vi "StepUI.vi"() -> ()   [LabVIEW 2015, in "StepNode.lvclass"]
doc: "Copyright 2017 National Instruments Corporation\n\nLicensed under the Apache License, Version 2.0 (the \"License\"); you may not use this file except in compliance with the License. You may obtain a copy of the License at http://www.apache.org/licenses/LICENSE-2.0\nUnless required by applicable law or agreed to in writing, software distributed under the License is distributed on an \"AS IS\" BASIS, WITHOUT WARRANTIES OR CONDITIONS OF ANY KIND, either express or implied. See the License for the specific language governing permissions and limitations under the License."
uses:
  StepNode.lvclass
  <vilib>/NI/Configuration Framework/Node/NodeRef.ctl
  <vilib>/NI/Configuration Framework/Node/NISE_CEF_Node.lvclass
  <vilib>/NI/AMC/Message Queue.ctl
  <vilib>/NI/AMC/Message.ctl
  <vilib>/NI/Tools/Keyed Array/KeyedArray.ctl
  <vilib>/NI/Configuration Framework/Node/UserEventRef.ctl
  <vilib>/NI/Configuration Framework/Controls/EventCluster.ctl
  Prototype/classes/Step/UI/Controls/Step UI Main Parameters.ctl
  <vilib>/NI/Configuration Framework/Node/NISE_CEF_Node.lvclass/NISE_CEF_Node.ctl
  <vilib>/NI/Configuration Framework/Node/ReadParent.vi
  <vilib>/NI/AMC/Create Single Message.vi
  <vilib>/NI/AMC/Update Message Routing Info.vi
  <vilib>/NI/AMC/Send Message.vi
  Prototype/classes/Step/UI/Step UI.lvclass
  <vilib>/NI/AMC/AMC.lvlib
  <vilib>/NI/Configuration Framework/NISE_CEF_TreeControl.lvlib
  <vilib>/NI/Tools/Keyed Array/Tools_KeyedArray.lvlib
panel:
  in  "Down Button":bool
  in  "Up Button":bool
  out "Step Details":cluster{"Type":string, "Version":string}
  in  "General Parameters":cluster{"Skip?":bool, "Step Name":string}
  in  "user event":T1
  in  "main queue":T2
  in  "node ref":T3
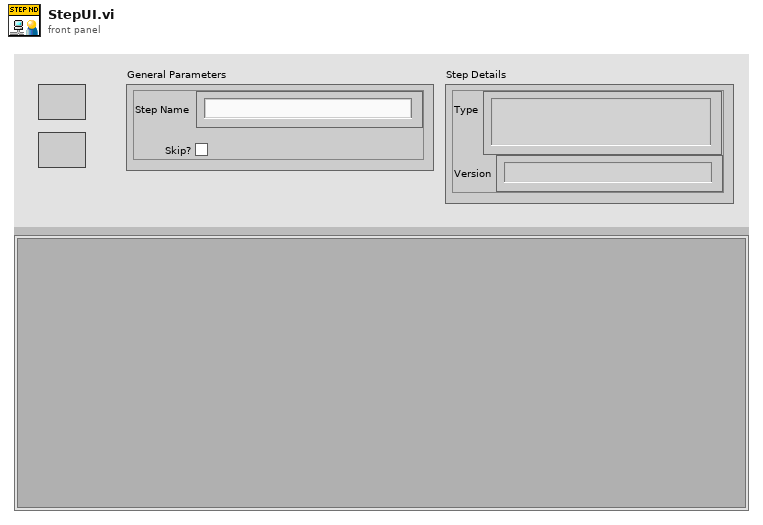
[diagram p1: front panel]
types:
  T1 = typedef "NISE_CEF_Node.lvclass/UserEventRef.ctl" = refnum<user-event>
  T2 = typedef "AMC.lvlib/Message Queue.ctl" = refnum<queue>
  T3 = typedef "NISE_CEF_Node.lvclass/NodeRef.ctl" = refnum<data-value>
  T4 = typedef "Step UI.lvclass/Step UI Main Parameters.ctl" = cluster{"main queue":T2, "data value reference":refnum<data-value>, "user event":T1}
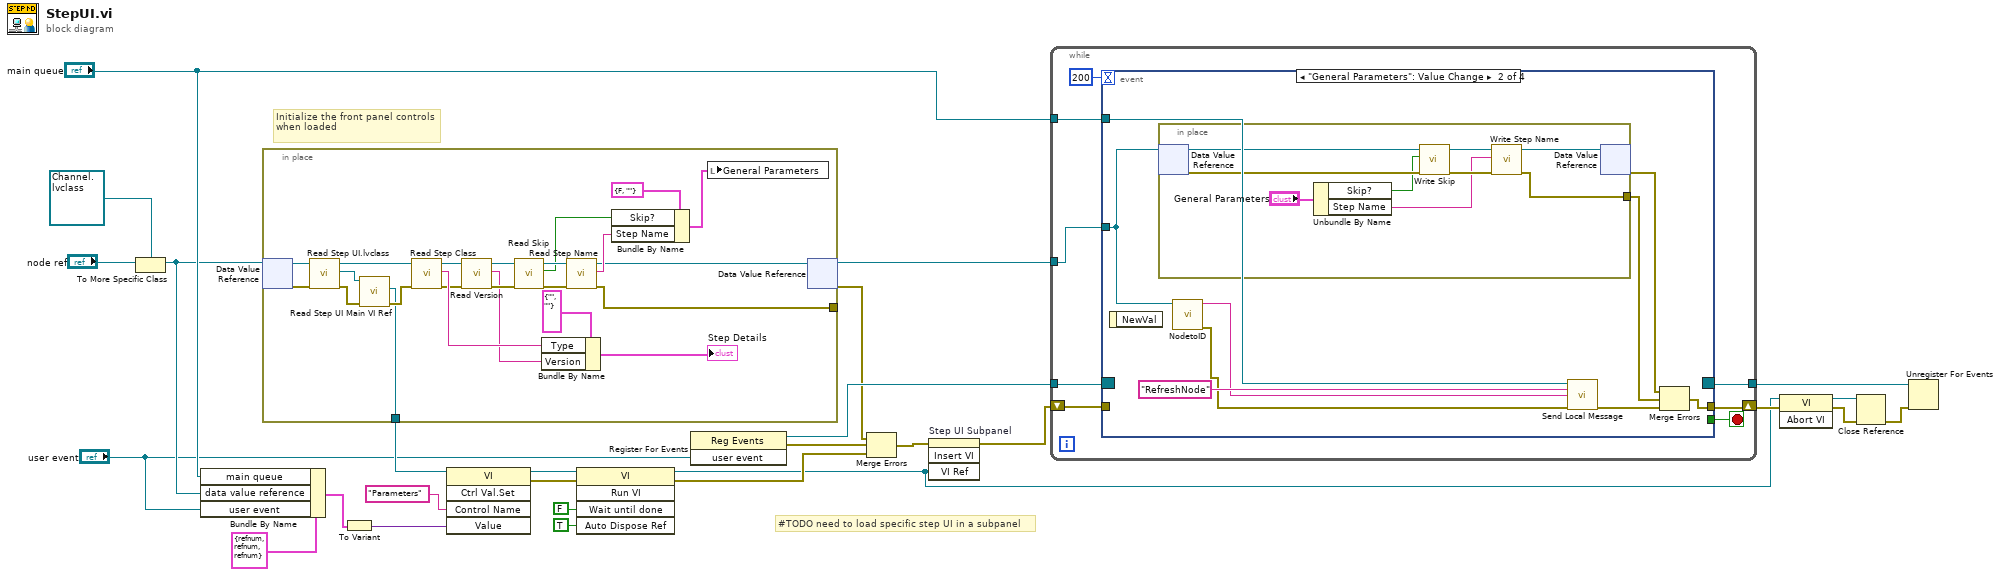
[diagram p0: block diagram]
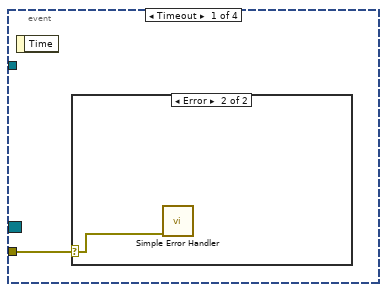
[diagram p2: hidden frame]
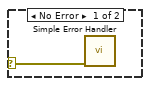
[diagram p3: hidden frame]
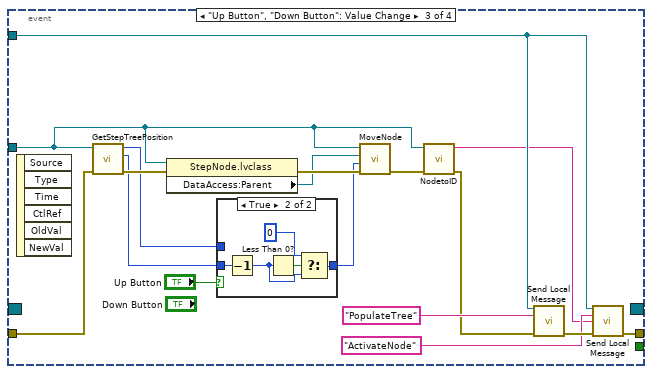
[diagram p4: hidden frame]
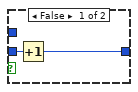
[diagram p5: hidden frame]
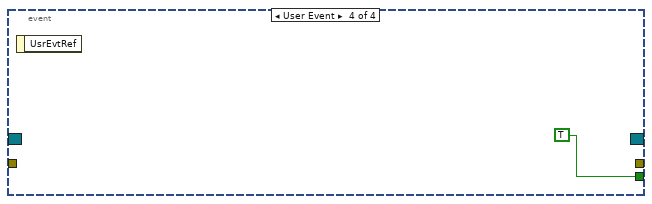
[diagram p6: hidden frame]
diagram:
  # "Initialize the front panel controls when loaded"
  # "#TODO need to load specific step UI in a subpanel"
  n1 = To More Specific Class(target class=refnum<data-value> refnum ("data value reference"), reference="node ref") -> (specific class reference=w4:refnum<data-value>)  [unwired: 1 in, 1 out]
  n2 = Bundle By Name(cluster=T4 {"main queue"=refnum, "data value reference"=refnum, "user event"=refnum}, "main queue"="main queue", "data value reference"=w4, "user event"="user event") -> (w2:T4)
  n3 = in-place {
    in-place-border: [w45] -> _
    in-place-border: [w28] -> w17
    n4 = in-place-dvr #1(w4) -> (w33:refnum<class "StepNode.lvclass">, w48:errorcluster)
    n5 = call-dynamic "Read Step UI.lvclass.vi"("error in (no error)"=w48, "StepNode in"=w33) -> ("error out"=w30:errorcluster, "Step UI.lvclass"=w31:refnum<class "Step UI.lvclass">, "StepNode out"=w32:refnum<class "StepNode.lvclass">)  [unwired: 7 in]
    n6 = call-dynamic "Read Step UI Main VI Ref.vi"("error in (no error)"=w30, "Step UI in"=w31) -> ("error out"=w29:errorcluster, "Step UI Main VI Ref"=w28:refnum<vi>)  [unwired: 7 in, 1 out]
    n7 = call-dynamic "Read Step Class.vi"("error in (no error)"=w29, "StepNode in"=w32) -> ("error out"=w35:errorcluster, "Step Class"=w47:string, "StepNode out"=w36:refnum<class "StepNode.lvclass">)  [unwired: 7 in]
    n8 = call-dynamic "Read Version.vi"("error in (no error)"=w35, "StepNode in"=w36) -> ("error out"=w40:errorcluster, "Version"=w38:string, "StepNode out"=w39:refnum<class "StepNode.lvclass">)  [unwired: 7 in]
    n9 = call-dynamic "Read Skip.vi"("error in (no error)"=w40, "StepNode in"=w39) -> ("error out"=w46:errorcluster, "Skip"=w42:bool, "StepNode out"=w44:refnum<class "StepNode.lvclass">)  [unwired: 7 in]
    n10 = Bundle By Name(cluster=cluster{"Type":string, "Version":string} {"Type"="", "Version"=""} ("Step Details"), "Type"=w47, "Version"=w38) -> (→"Step Details":cluster{"Type":string, "Version":string})
    n11 = call-dynamic "Read Step Name.vi"("error in (no error)"=w46, "StepNode in"=w44) -> ("error out"=w45:errorcluster, "Step Name"=w41:string, "StepNode out"=w37:refnum<class "StepNode.lvclass">)  [unwired: 7 in]
    n12 = Bundle By Name(cluster=cluster{"Skip?":bool, "Step Name":string} {"Skip?"=FALSE, "Step Name"=""} ("General Parameters"), "Skip?"=w42, "Step Name"=w41) -> (w43:cluster{"Skip?":bool, "Step Name":string})
    n13 = local write "General Parameters"(w43) -> ()
    n14 = in-place-dvr #1(w37) -> (w27:refnum<data-value>, w20:errorcluster)
  }
  n15 = To Variant(anything=w2) -> (Variant=w7:variant)
  n16 = invoke class="VI" method="Ctrl Val.Set"(reference=w17, "Control Name"="Parameters", "Value"=w7) -> (reference out=w9:refnum<vi>, error out=w6:errorcluster)  [unwired: 2 in, 3 out]
  n17 = invoke class="VI" method="Run VI"(reference=w9, error in=w6, "Wait until done"=FALSE ("Wait Until Done"), "Auto Dispose Ref"=TRUE ("Auto Dispose Reference")) -> (reference out=w12:refnum<vi>, error out=w16:errorcluster)  [unwired: 1 in, 3 out]
  n18 = register-events("user event") -> (reference out=w26:refnum<event-registration>, error out=w21:errorcluster)  [unwired: 2 in]
  n19 = Merge Errors(w20, w21, w16) -> (w19:errorcluster)
  n20 = invoke on="Step UI Subpanel" class="SubPnl" method="Insert VI"(error in=w19, "VI Ref"=w12) -> (error out=w18:errorcluster)  [unwired: 2 in, 3 out]
  n21 = while {
    tunnel: w27 -> [w58]
    tunnel: "main queue" -> [w57]
    tunnel: w26 -> [w55]
    tunnel: [w54] -> w25
    shift-right: [w52] -> w24
    shift-left: w18 -> [w51]
    stop <- w53 stop-if-true
    n22 = event shown="[1] \"General Parameters\": Value Change" {
      selector: w55 -> [_ _ _ _]
      dyn-events: [_ _ _ _] -> w54
      timeout: 200 -> [_ _ _ _]
      tunnel: w58 -> [_ w68 w83 _]
      tunnel: w57 -> [_ w69 w86 _]
      tunnel: [_ _ _ TRUE] -> w53
      tunnel: [_ w65 w87 _] -> w52
      tunnel: w51 -> [w59 _ w96 _]
      event Timeout {
        n23 = event-data() -> ()  [unwired: 1 in, 1 out]
        n24 = case shown="Error" w59 {
          selector: w59 -> [w60 w61]
          frame No Error {
            n25 = call <vilib>:"Simple Error Handler.vi"("error in (no error)"=w60) -> ()  [unwired: 4 in, 5 out]
          }
          frame Error {
            n26 = call <vilib>:"Simple Error Handler.vi"("error in (no error)"=w61) -> ()  [unwired: 4 in, 5 out]
          }
        }
      }
      event "General Parameters": Value Change {
        n27 = event-data() -> ()  [unwired: 1 in, 1 out]
        n28 = in-place {
          in-place-border: [w74] -> w63
          n29 = in-place-dvr #2(w68) -> (w76:refnum<class "StepNode.lvclass">, w79:errorcluster)
          n30 = Unbundle By Name("General Parameters") -> ("Skip?"=w75:bool, "Step Name"=w71:string)
          n31 = call-dynamic "Write Skip.vi"("error in (no error)"=w79, "Skip"=w75, "StepNode in"=w76) -> ("error out"=w77:errorcluster, "StepNode out"=w73:refnum<class "StepNode.lvclass">)  [unwired: 7 in]
          n32 = call-dynamic "Write Step Name.vi"("error in (no error)"=w77, "Step Name"=w71, "StepNode in"=w73) -> ("error out"=w74:errorcluster, "StepNode out"=w72:refnum<class "StepNode.lvclass">)  [unwired: 7 in]
          n33 = in-place-dvr #2(w72) -> (w64:errorcluster)  [unwired: 1 out]
        }
        n34 = call <vilib>:"NodetoID.vi"("node ref"=w68) -> ("error out"=w62:errorcluster, "ID"=w67:string)  [unwired: 9 in]
        n35 = call <vilib>:"Send Local Message.vi"("message queue in"=w69, "message name"="RefreshNode" ("Message Name"), "message value"=w67, "error in"=w62) -> ("error out"=w66:errorcluster)  [unwired: 9 in, 2 out]
        n36 = Merge Errors(w64, w63, w66) -> (w65:errorcluster)
      }
      event "Up Button", "Down Button": Value Change {
        n37 = event-data() -> ()  [unwired: 1 in, 6 out]
        n38 = call "GetStepTreePosition.vi"("error in (no error)"=w96, "Node Reference in"=w83) -> ("error out"=w95:errorcluster, "TreeIndex"=w93:i32, "#Nodes"=w80:i32)  [unwired: 7 in]
        n39 = property class="StepNode.lvclass"(reference=w83, error in=w95) -> (error out=w94:errorcluster, "DataAccess:Parent"=w81:T3)  [unwired: 1 out]
        n40 = case shown="True" "Up Button" {
          tunnel: w93 -> [w98 w103]
          tunnel: [w97 w100] -> w90
          tunnel: w80 -> [_ _]
          frame False {
            n41 = Increment(x=w98) -> (x+1=w97:i32)
          }
          frame True {
            n42 = Decrement(x=w103) -> (x-1=w99:i32)
            n43 = Less Than 0?(x=w99) -> (x < 0?=w102:bool)
            n44 = Select(t=0 ("x"), s=w102, f=w99) -> (s? t:f=w100:i32)
          }
        }
        n45 = call <vilib>:"MoveNode.vi"("error in"=w94, "index"=w90, "new parent"=w81, "node"=w83) -> ("error out"=w91:errorcluster)  [unwired: 7 in]
        n46 = call <vilib>:"NodetoID.vi"("error in"=w91, "node ref"=w83) -> ("error out"=w84:errorcluster, "ID"=w82:string)  [unwired: 8 in]
        n47 = call <vilib>:"Send Local Message.vi"("message queue in"=w86, "message name"="PopulateTree", "error in"=w84) -> ("error out"=w89:errorcluster)  [unwired: 10 in, 2 out]
        n48 = call <vilib>:"Send Local Message.vi"("message queue in"=w86, "message name"="ActivateNode", "message value"=w82, "error in"=w89) -> ("error out"=w87:errorcluster)  [unwired: 9 in, 2 out]
      }
      event User Event {
        n49 = event-data() -> ()  [unwired: 1 in, 1 out]
      }
    }
  }
  n50 = invoke class="VI" method="Abort VI"(reference=w12, error in=w24) -> (reference out=w10:refnum<vi>, error out=w13:errorcluster)  [unwired: 1 in, 1 out]
  n51 = Close Reference(reference=w10, error in (no error)=w13) -> (error out=w11:errorcluster)
  n52 = Unregister For Events(event registration refnum=w25, error in=w11) -> ()  [unwired: 1 out]
